vi "Cast 2D to 1D.vi"(1 "1D size":i32, 2 "2D Synchronous Monkeys":T1[][](array[typedef])) -> (0 "1D Synchronous Monkeys":T1[](array[typedef]))   [LabVIEW 2020, in "Tamer.lvlib" / "Tamer.lvclass"]
uses:
  Tamer.lvclass
  Monkey Summary.ctl
  Run Utilities/TypeDefs/Monkey Status.ctl
  Link Chain GUI.ctl
  Run Utilities/Run Utilities.lvlib
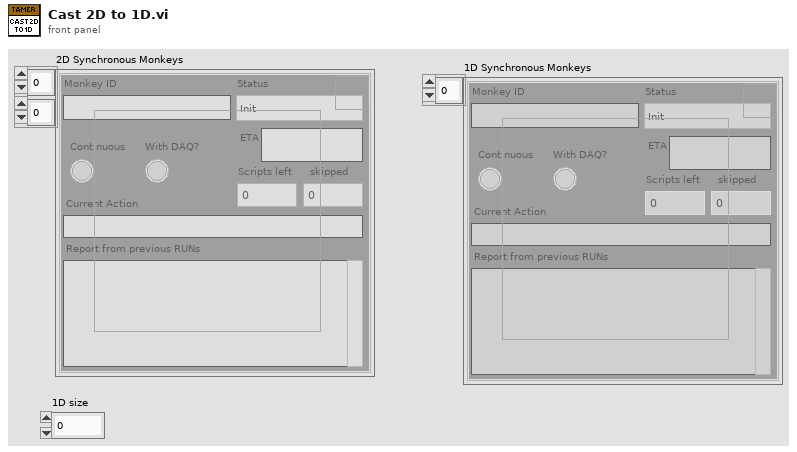
[diagram p1: front panel]
types:
  T1 = typedef "Tamer.lvlib/Tamer.lvclass/Monkey Summary.ctl" = cluster{"Color":u32, "Status":T2, "Continuous":bool, "Scripts left":u32, "Scripts skipped":u32, "ETA":string, "Current Action":string, "Report from previous RUNs":string, "Monkey ID":string, "With DAQ?":bool, "Linked?":T3, "Paused":bool}
  T2 = typedef "TALOS.lvlib/Run Utilities.lvlib/Monkey Status.ctl" = enum16{"Init", "Paused", "Ongoing", "Stopped", "Finished (no errors)", "Finished (with errors)"}
  T3 = typedef "Tamer.lvlib/Tamer.lvclass/Link Chain GUI.ctl" = bool
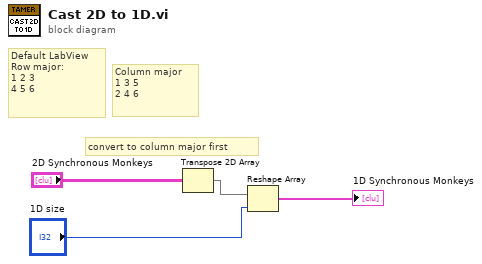
[diagram p0: block diagram]
diagram:
  # "Column major\n1 3 5\n2 4 6"
  # "Default LabView\nRow major:\n1 2 3\n4 5 6"
  # "convert to column major first"
  n1 = Transpose 2D Array(2D array="2D Synchronous Monkeys") -> (transposed array=w1:T1[][])
  n2 = Reshape Array(w1, "1D size") -> (→"1D Synchronous Monkeys":T1[])
